vi "Get Current Position.vi"(8 "error in (no error)":errorcluster, 11 "SIM Motion Controller in":refnum<class "Fine SIM Motion Controller.lvclass">) -> (0 "error out":errorcluster, 2 "Current Position":dbl, 3 "SIM Motion Controller out":refnum<class "Fine SIM Motion Controller.lvclass">)   [LabVIEW 2022 SP3, in "Fine SIM Motion Controller.lvclass"]
uses:
  Fine SIM Motion Controller.lvclass
  C:/Stage-Work/MAS/Axis Objects/Motion Controller/Parent SIM Motion Controller.lvclass
  Motion Controller/Parent SIM Motion Controller.lvclass/Parent SIM Motion Controller.ctl
  Motion Controller/Accessors/Read Sim Axis Data.vi
  Motion Controller/Accessors/Write Sim Axis Data.vi
  Fine SIM Motion Controller.lvclass/Fine SIM Motion Controller.ctl
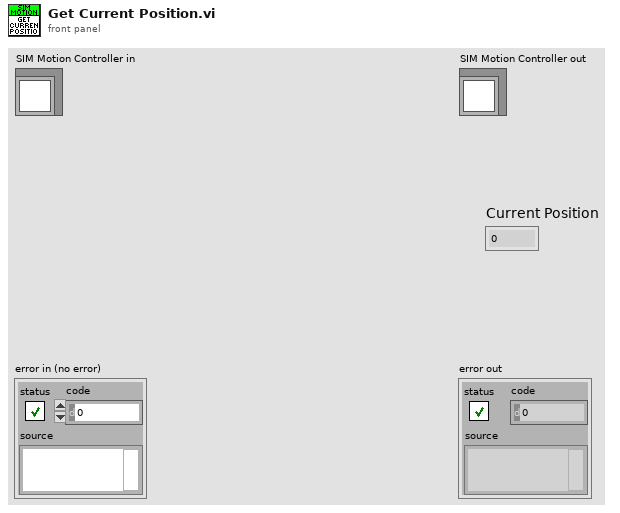
[diagram p1: front panel]
types:
  T1 = typedef "Parent SIM Motion Controller.lvclass/Axis Data.ctl" = cluster{"Axis Parameters":T2, "Axis Settings":T3, "Time Stamp":timestamp}
  T2 = typedef "Parent SIM Motion Controller.lvclass/Axis Parameters.ctl" = cluster{"Moving":bool, "Homed":bool, "Desired Position":dbl, "Current Positon":dbl, "Current Speed":dbl}
  T3 = typedef "Parent SIM Motion Controller.lvclass/Axis Settings.ctl" = cluster{"Speed":dbl, "Acceleration":dbl}
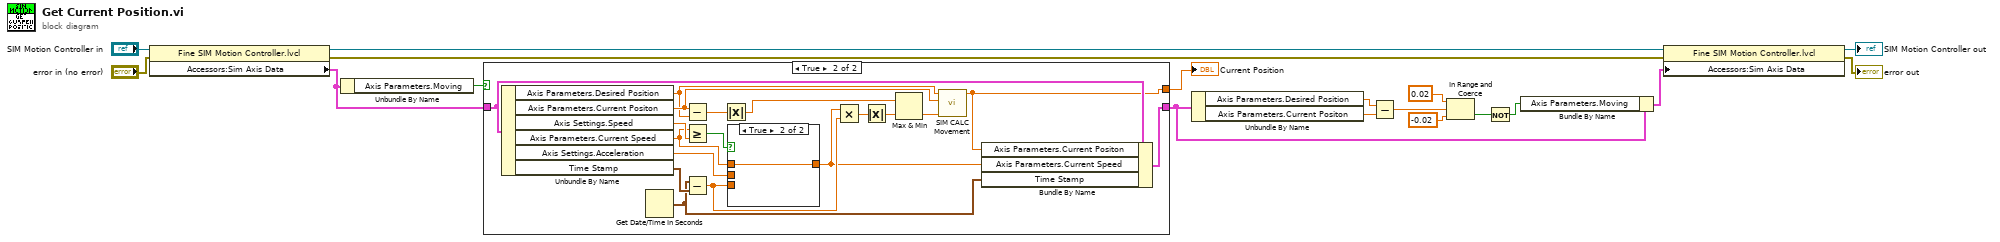
[diagram p0: block diagram]
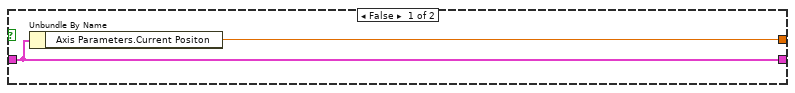
[diagram p2: hidden frame]
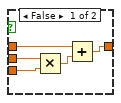
[diagram p3: hidden frame]
diagram:
  n1 = property class="Fine SIM Motion Controller.lvcl"(reference="SIM Motion Controller in", error in="error in (no error)") -> (reference out=w17:refnum<class "Fine SIM Motion Controller.lvclass">, error out=w13:errorcluster, "Accessors:Sim Axis Data"=w10:T1)
  n2 = Unbundle By Name(w10) -> ("Axis Parameters.Moving"=w11:bool)
  n3 = case shown="True" w11 {
    tunnel: w10 -> [w20 w38]
    tunnel: [w20 w37] -> w2
    tunnel: [w19 w29] -> w14
    frame False {
      n4 = Unbundle By Name(w20) -> ("Axis Parameters.Current Positon"=w19:dbl)
    }
    frame True {
      n5 = Unbundle By Name(w38) -> ("Axis Parameters.Desired Position"=w26:dbl, "Axis Parameters.Current Positon"=w27:dbl, "Axis Settings.Speed"=w34:dbl, "Axis Parameters.Current Speed"=w33:dbl, "Axis Settings.Acceleration"=w32:dbl, "Time Stamp"=w30:timestamp)
      n6 = Get Date/Time In Seconds() -> (seconds since 1Jan1904=w28:timestamp)
      n7 = Subtract(x=w27, y=w26) -> (x-y=w25:dbl)
      n8 = Greater Or Equal?(x=w33, y=w34) -> (x >= y?=w35:bool)
      n9 = Subtract(x=w28, y=w30) -> (x-y=w36:dbl)
      n10 = Absolute Value(x=w25) -> (abs(x)=w23:dbl)
      n11 = case shown="True" w35 {
        tunnel: [w39 w44] -> w31
        tunnel: w33 -> [w40 w44]
        tunnel: w36 -> [w43 _]
        tunnel: w32 -> [w42 _]
        frame False {
          n12 = Multiply(x=w42, y=w43) -> (x*y=w41:dbl)
          n13 = Add(x=w40, y=w41) -> (x+y=w39:dbl)
        }
        frame True {
        }
      }
      n14 = Multiply(x=w31, y=w36) -> (x*y=w24:dbl)
      n15 = Absolute Value(x=w24) -> (abs(x)=w22:dbl)
      n16 = Max & Min(x=w23, y=w22) -> (min(x,y)=w21:dbl)  [unwired: 1 out]
      n17 = call "SIM CALC Movement.vi"("New Distance"=w21, "Current"=w27, "Desired"=w26) -> ("New Current"=w29:dbl)  [unwired: 8 in]
      n18 = Bundle By Name(cluster=w38, "Axis Parameters.Current Positon"=w29, "Axis Parameters.Current Speed"=w31, "Time Stamp"=w28) -> (w37:T1)
    }
  }
  "Current Position" <- w14
  n19 = Unbundle By Name(w2) -> ("Axis Parameters.Desired Position"=w8:dbl, "Axis Parameters.Current Positon"=w7:dbl)
  n20 = Subtract(x=w8, y=w7) -> (x-y=w6:dbl)
  n21 = In Range and Coerce(upper limit=0.02, x=w6, lower limit=-0.02) -> (In Range?=w3:bool)  [unwired: 1 out]
  n22 = Not(x=w3) -> (.not. x?=w9:bool)
  n23 = Bundle By Name(cluster=w2, "Axis Parameters.Moving"=w9) -> (w1:T1)
  n24 = property class="Fine SIM Motion Controller.lvcl"(reference=w17, error in=w13, "Accessors:Sim Axis Data"=w1) -> (reference out=→"SIM Motion Controller out":refnum<class "Fine SIM Motion Controller.lvclass">, error out=→"error out":errorcluster)
